vi "init.vi"(8 "error in (no error)":errorcluster, 11 "StiffnessCalculator in":refnum<class "StiffnessCalculator.lvclass">) -> (0 "error out":errorcluster, 3 "StiffnessCalculator out":refnum<class "StiffnessCalculator.lvclass">)   [LabVIEW 2015, in "StiffnessCalculator.lvclass"]
uses:
  StiffnessCalculator.lvclass
  Configuration/StiffnessCalculator.ctl
  ConfigurationThisComponent/ConfigurationThisComponent.lvclass
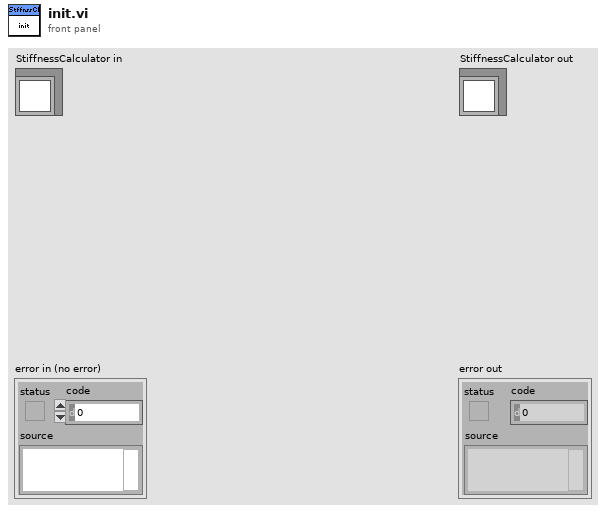
[diagram p1: front panel]
types:
  T1 = typedef "StiffnessCalculator.ctl" = cluster{"Forces in Stiffness Summary":dbl[unit][]}
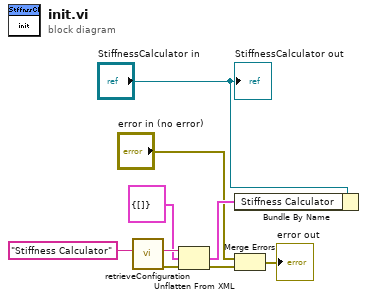
[diagram p0: block diagram]
diagram:
  n1 = call "retrieveConfiguration.vi"("configName"="Stiffness Calculator") -> ("error out"=w7:errorcluster, "xmlConfig"=w6:string)  [unwired: 8 in, 1 out]
  n2 = Unflatten From XML(xml string=w6, type=T1 {"Forces in Stiffness Summary"=[]} ("Stiffness Calculator"), error in (no error)=w7) -> (value=w3:T1, error out=w9:errorcluster)
  n3 = Bundle By Name(cluster="StiffnessCalculator in", "Stiffness Calculator"=w3) -> ()  [unwired: 1 out]
  n4 = Merge Errors("error in (no error)", w9) -> (→"error out":errorcluster)
  "StiffnessCalculator out" <- "StiffnessCalculator in"
